vi "Nominal Value Write Single.vi"(8 "error in":errorcluster, 9 "Channel Index":i32=1, 10 "Nominal Value":dbl, 11 "Nominal Value in":refnum<class "Nominal Value.lvclass">) -> (0 "error out":errorcluster, 3 "Nominal Value out":refnum<class "Nominal Value.lvclass">)   [LabVIEW 2023, in "Nominal Value.lvclass"]
uses:
  Nominal Value.lvclass
  <vilib>/ADAS Replay HIL/Channels/Tag Wrapper/Tag Wrapper.lvlib
  <vilib>/ADAS Replay HIL/Channels/Tag Wrapper/Polymorphic/Write Channel (Double).vi
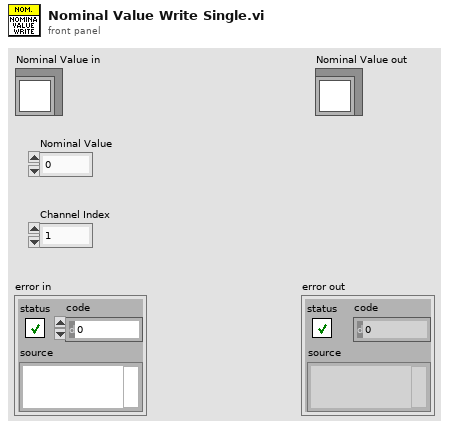
[diagram p1: front panel]
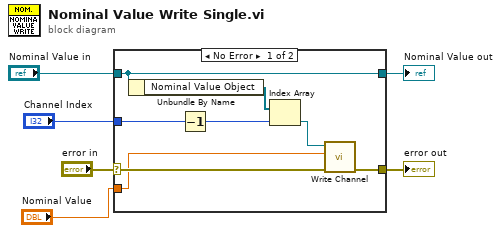
[diagram p0: block diagram]
diagram:
  n1 = case shown="No Error" "error in" {
    selector: "error in" -> [w14 w15]
    tunnel: [w13 w15] -> w5
    tunnel: [w11 w16] -> w2
    tunnel: "Nominal Value in" -> [w11 w16]
    tunnel: "Nominal Value" -> [w12 _]
    tunnel: "Channel Index" -> [w8 _]
    frame No Error {
      n2 = Unbundle By Name(w11) -> ("Nominal Value Object"=w10:refnum<k21>[])
      n3 = Decrement(x=w8) -> (x-1=w7:i32)
      n4 = Index Array(array=w10, index=w7) -> (element=w9:refnum<k21>)
      n5 = call-poly <vilib>:"Write Channel.vi"("error in"=w14, "Value to Write"=w12, "ADAS HIL Channel in"=w9) -> ("error out"=w13:errorcluster)  [unwired: 6 in, 2 out]
    }
    frame Error {
    }
  }
  "error out" <- w5
  "Nominal Value out" <- w2
